vi "Actor Decorator.vi"(10 "Actor":refnum<class "Actor.lvclass">, 11 "Self Actor in":refnum<class "Self Actor.lvclass">) -> (3 "Self Actor out":refnum<class "Self Actor.lvclass">)   [LabVIEW 2021, in "AAM.lvlib" / "Self Actor.lvclass"]
uses:
  Self Actor.lvclass
  Actor/Actor.lvclass
  Self Actor.lvclass/Self Actor.ctl
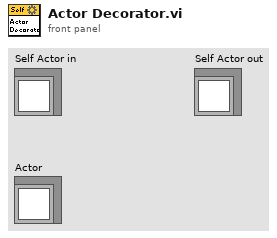
[diagram p1: front panel]
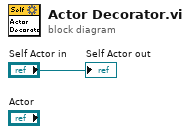
[diagram p0: block diagram]
diagram:
  "Self Actor out" <- "Self Actor in"
